vi "DI_FAST queue.vi"(5 "object":string="AZ1", 6 "DI state table":T1[](array[typedef]), 7 "date/time string":string, 9 "discret parameters":bool[](array[boolean]), 10 "DI table":string[](array[string]), 11 "DI_FAST_msg":refnum<queue>) -> ()   [LabVIEW 2019, in "Inputs.lvlib"]
uses:
  Inputs.lvlib
  Ctl/Parameter State.ctl
  Database/PostgreSQL.lvlib
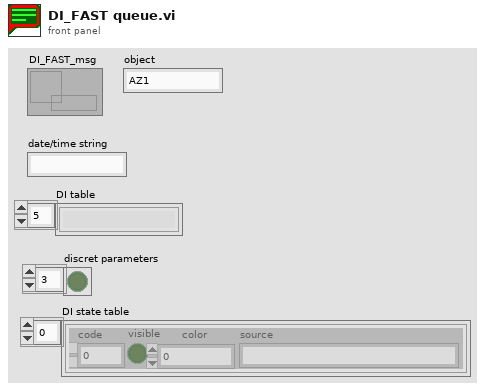
[diagram p1: front panel]
types:
  T1 = typedef "Inputs.lvlib/Parameter State.ctl" = cluster{"code":i32, "visible":bool, "color":u32, "source":string}
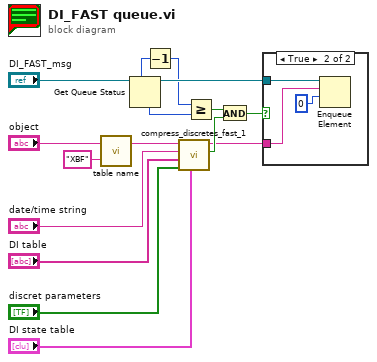
[diagram p0: block diagram]
diagram:
  n1 = call "table name.vi"("postfix"="XBF", "object name"="object") -> ("table name"=w1:string)  [unwired: 1 in]
  n2 = Get Queue Status(queue="DI_FAST_msg") -> (queue out=w15:refnum<queue>, max queue size=w13:i32, # elements in queue=w14:i32)  [unwired: 2 in, 5 out]
  n3 = Decrement(x=w13) -> (x-1=w12:i32)
  n4 = call "compress_discretes_fast_1.vi"("DI state table"="DI state table", "discret parameters"="discret parameters", "DI table"="DI table", "date/time string"="date/time string", "table"=w1) -> ("Data to write"=w9:bool, "parameters"=w8:string)  [unwired: 5 in]
  n5 = Greater Or Equal?(x=w12, y=w14) -> (x >= y?=w11:bool)
  n6 = And(x=w11, y=w9) -> (x .and. y?=w10:bool)
  n7 = case shown="True" w10 {
    tunnel: w15 -> [_ w18]
    tunnel: w8 -> [_ w17]
    frame False {
    }
    frame True {
      n8 = Enqueue Element(queue=w18, element=w17, timeout in ms (-1)=0) -> ()  [unwired: 1 in, 3 out]
    }
  }
